vi "Measure Acoustic Frequency Response.vi"() -> ()   [LabVIEW 2022 SP3]
uses:
  <vilib>/addons/_NISVFA/_Generation/Signal Generation/SV Signal/SV Signal.lvclass/SV Signal.ctl
  <vilib>/DAQmx/write.llb/DAQmx Write (Analog Wfm 1Chan NSamp).vi
  <vilib>/DAQmx/read.llb/DAQmx Read (Analog 1D Wfm NChan NSamp).vi
  <vilib>/addons/Sound and Vibration/svt_Level/SVL AC & DC Level (Time) (1 Ch).vi
  <vilib>/addons/_NISVFA/_Generation/Signal Generation/SV Signal/Write Leading Synchronization Pulse Enable.vi
  <vilib>/addons/_NISVFA/_Generation/Signal Generation/SV Signal/Read Total Samples.vi
  <vilib>/addons/_NISVFA/_Shared subVIs/Common/svc_Get SV Channel Info.vi
  <vilib>/Analysis/baseanly.llb/Mean.vi
  <vilib>/Analysis/baseanly.llb/Mean (DBL).vi
  <vilib>/addons/_NISVFA/_Shared subVIs/Windowing/svfa_Scaled Time Domain Window (Array).vi
  <vilib>/addons/_NISVFA/_Generation/Signal Generation/SV Signal/Calculate Number of Remaining Samples.vi
  <vilib>/addons/_NISVFA/_Shared subVIs/Common/svc_Unit Label to Engineering Units.vi
  <vilib>/addons/_NISVFA/_Shared subVIs/Common/svc_Engineering Units to Unit Label.vi
  <vilib>/addons/_NISVFA/_Spectrum Processing/subVIs/svfa_Spectrum Info Window to windowTd Type Def.vi
  <vilib>/Analysis/4window.llb/Force Window.vi
  <vilib>/Analysis/4window.llb/Force Window (DBL).vi
  <vilib>/Analysis/4window.llb/Exponential Window.vi
  <vilib>/Analysis/4window.llb/Exponential Window (DBL).vi
  <vilib>/addons/_NISVFA/_Generation/Signal Generation/SV Discrete Sweep/SV Discrete Sweep.lvclass
  C:/Program Files/NI/LVAddons/nisvt/1/vi.lib/addons/_NISVFA/_Generation/Signal Generation/SV Signal/SV Signal.lvclass
  C:/Program Files/NI/LVAddons/nisvt/1/vi.lib/addons/_NISVFA/_Generation/Signal Generation/SV Function/SV Function.lvclass
  <vilib>/addons/_NISVFA/_Generation/Signal Generation/SV Discrete Sweep/Configure Frequency Sweep at Constant Amplitude.vi
  <vilib>/addons/_NISVFA/_Generation/Signal Generation/SV Signal/Write Ramp Parameters.vi
  <vilib>/addons/_NISVFA/_Generation/Signal Generation/SV Signal/Write Measurement Duration.vi
  <vilib>/addons/_NISVFA/_Generation/Signal Generation/SV Function/Write Measurement Cycles.vi
  <vilib>/addons/_NISVFA/_Generation/Signal Generation/SV Signal/Write Pre-Measurement Settling Duration.vi
  <vilib>/addons/_NISVFA/_Generation/Signal Generation/SV Function/Write Pre-Measurement Settling Cycles.vi
  <vilib>/addons/_NISVFA/_Generation/Signal Generation/SV Signal/Write Sample Rate.vi
  <vilib>/addons/_NISVFA/_Generation/Signal Generation/SV Signal/Read Generation State.vi
  <vilib>/addons/_NISVFA/_Generation/Signal Generation/SV Signal/Read System Timing Model.vi
  <vilib>/DAQmx/create/channels.llb/DAQmx Create Channel (AO-Voltage-Basic).vi
  <vilib>/DAQmx/configure/timing.llb/DAQmx Timing (Sample Clock).vi
  <vilib>/DAQmx/create/channels.llb/DAQmx Create Channel (AI-Sound Pressure-Microphone).vi
  <vilib>/DAQmx/configure/trigger.llb/DAQmx Start Trigger (Digital Edge).vi
  <vilib>/DAQmx/miscellaneous.llb/DAQmx Fill In Error Info.vi
  <vilib>/addons/_NISVFA/_Shared subVIs/Data Objects/Waveforms (DBL)/SV Read Next Measurement Data.vi
  <vilib>/addons/_NISVFA/_Shared subVIs/Common/svc_Get Window Info.vi
  <vilib>/Analysis/0measdsp.llb/Scaled Time Domain Window.vi
  <vilib>/Analysis/0measdsp.llb/Scaled Time Domain Window (DBL).vi
  <vilib>/Utility/error.llb/Error Cluster From Error Code.vi
  <vilib>/Analysis/baseanly.llb/Std Deviation and Variance.vi
  <vilib>/addons/_NISVFA/_Shared subVIs/Common/svc_Caller VI Returned in Error Source.vi
  <vilib>/addons/_NISVFA/_Spectrum Processing/SVFA Extract Single Tone Information (Waveform) (1 Ch).vi
  <vilib>/addons/_NISVFA/_Generation/Signal Generation/SV Signal/SV Signal.lvclass
  <resource>/objmgr/daqmx.rc
  <vilib>/addons/_NISVFA/_Shared subVIs/Data Objects/Waveforms (DBL)/Waveforms (N Ch).lvclass
  Program Files/NI/LVAddons/nisvt/1/examples/Sound and Vibration/SoundVib_Audio Examples.lvlib
  C:/Program Files/NI/LVAddons/nisvt/1/vi.lib/addons/_NISVFA/_Generation/Signal Generation/SV Sinusoid/SV Sinusoid.lvclass
  C:/Program Files/NI/LVAddons/nisvt/1/vi.lib/addons/_NISVFA/_Generation/Signal Generation/SV Discrete Sweep/SV Discrete Sweep.lvclass
panel:
  in  "Tab Control":enum32{"Time Domain", "Frequency Response"}(tab)=enum."Frequency Response"
  out "Waveform Graph":waveform(dbl)[](graph)=[{"t0"=timestamp(3812131384.799704 s since 1904-01-01), "dt"=1.9531249997269942e-05, "Y"=array[65939 elements], "attributes"=variant("NI_ChannelName"=variant(string "PXI1Slot2/ai0"), "NI_UnitDescription"=variant(string "Pascals"), "NI_dBReference"=variant(dbl 2e-05))}]
  out "Frequency Response":cluster{"X":dbl[], "Y":dbl[]}[](graph)=[{"X"=[10000.16250895643, 9300.551526537287, 8661.743392898796, 8076.990528350523, 7511.01433955411, 6991.165488423958, 6505.639524722646, 6059.649462837425, 5638.791827094052, 5251.483585942611, 4886.97833468438, 4567.629353940343, 4235.587558900483, 3936.8799678267396, 3676.0502040083957, 3418.4961516219546, 3182.8940845825587, 2961.9472023846033, 2757.249181768, 2566.403361400688, 2390.9470010062046, 2227.3394374433965, 2082.105166052262, 1927.4899981379963, 1795.2096498866752, 1671.116877761199, 1555.7617010555734, 1449.1771890209513, 1348.0642866026876, 1254.8715887027722, 1168.0622703473373, 1087.8906461237023, 1012.6424477531147, 942.8434270641828, 877.7564318056318, 816.9815108543755, 760.5623490709717, 708.309347567948, 659.4701187376695, 613.4296280137033, 571.3471132565072, 531.9637387870528, 495.24552739107736, 460.92109135700946, 429.09771808303145, 399.4620806680938, 371.8621259333098, 346.29727087738263, 322.46744887340316, 300.0397070573367], "Y"=[3.6256571566682783, -2.842824229562748, -0.08960303155444534, 2.249095345066365, 2.6453221558194495, 1.950185415035666, 1.243543034377954, -0.04093683877364576, 0.8379919469408734, 2.1848997103980627, 4.7478488049488305, 4.19605617553053, 5.612574046766889, 4.678952312370798, 4.014509980034741, 4.073090913593083, 4.332476772799007, 3.705298472623842, 1.6367797061942184, 4.064856703686522, 6.533918167683063, 5.093011293640562, 5.133330197154078, 4.011026255125055, 4.150393597006224, 4.30040032146349, 3.6036557635303956, 2.3710549475225817, 2.153214192355483, 2.56247383137912, 2.1421046081265924, 1.774553410980341, 0.05571083822585535, -1.5941096436671836, -1.5865003010327725, -1.8405935524517862, -1.9548534646079687, -1.8198185489247807, -1.9637495562133325, -3.3689527326194812, -3.271589837421542, -2.786050740963142, -2.6451973343748936, -2.077662686783256, -1.678738111514333, -1.682666406364262, -1.9245802060296682, -2.3869103430534615, -3.5810743320318554, -4.371652550879365]}, {"X"=[10000.16250895643, 9300.551526537287, 8661.743392898796, 8076.990528350523, 7511.01433955411, 6991.165488423958, 6505.639524722646, 6059.649462837425, 5638.791827094052, 5251.483585942611, 4886.97833468438, 4567.629353940343, 4235.587558900483, 3936.8799678267396, 3676.0502040083957, 3418.4961516219546, 3182.8940845825587, 2961.9472023846033, 2757.249181768, 2566.403361400688, 2390.9470010062046, 2227.3394374433965, 2082.105166052262, 1927.4899981379963, 1795.2096498866752, 1671.116877761199, 1555.7617010555734, 1449.1771890209513, 1348.0642866026876, 1254.8715887027722, 1168.0622703473373, 1087.8906461237023, 1012.6424477531147, 942.8434270641828, 877.7564318056318, 816.9815108543755, 760.5623490709717, 708.309347567948, 659.4701187376695, 613.4296280137033, 571.3471132565072, 531.9637387870528, 495.24552739107736, 460.92109135700946, 429.09771808303145, 399.4620806680938, 371.8621259333098, 346.29727087738263, 322.46744887340316, 300.0397070573367], "Y"=[0.014701549353104379, -0.03010901811941409, -0.0008149891758433986, -0.01724816607104709, -0.08804020536385895, 0.01171395282562733, -0.06632787060085114, -0.04128864064776648, -0.07708491466250654, -0.08538230980682754, 0.016481405604758487, -0.09831386011585251, -0.06731733883329304, -0.05245900086451385, 0.0012408175248640669, -0.07911554256372134, -0.10448091462567502, -0.03663756866557915, -0.08784017146392609, -0.08762859004910031, -0.023736243865102133, -0.0998077707827952, -0.05902392827547197, -0.14121406472839934, -0.1430330467707847, -0.1365549874396703, -0.13768685833752312, 0.05845974901477882, -0.08207883122647797, 0.034785537244882064, 0.3688104071747212, -0.05473682476494158, -0.030278179903617787, -0.13770022107713525, -0.07549590799892826, -0.04249834403098171, -0.16743475112056583, -0.20813210450439237, -0.09842685052319, -0.6864074560918922, -1.186238820840597, -0.1257540797947951, -0.040259662661179564, -0.07570918672218777, -0.10234120140370741, -0.5050386115903533, -0.6397558977539762, -0.04161640760409843, -0.07888582122962143, -2.3725881843457106]}]
  in  "sweep settings":T1(tab)=enum."EQ Settings"
  in  "speaker excitation channel":tag="PXI1Slot2/ao0"
  in  "microphone response channel":tag="PXI1Slot2/ai0"
  in  "sensor sensitivity [mV/Pa]":dbl=50.0
  in  "number of steps":i32=50 min=1
  in  "amplitude":dbl=94.0 format="%.2p dBSPL"
  in  "frequency spacing":enum16{"Linear", "Logarithmic"}(ring)=enum."Logarithmic"
  in  "sweep range":cluster{"start":dbl, "stop":dbl}={"start"=10000.0, "stop"=300.0} {"stop" min=0.0 format="%.2f"; "start" min=0.0 format="%.2f"}
  in  "output voltage ratio":dbl=3.394 format="%#_g Pa/V"
  in  "EQ Action":T2(ring)=enum."Load and Apply EQ"
  in  "EQ File":path=path "C:/dev/digital-microphone/test/EQ_test.csv"
  in  "measurement":cluster{"time":dbl, "cycles":dbl}={"time"=0.001, "cycles"=25.0} {"cycles" min=5.0 max=1000.0 step=1.0; "time" min=0.0 max=5.0 step=0.0001 format="%.3f s"}
  in  "settling":cluster{"time":dbl, "cycles":dbl}={"time"=0.0, "cycles"=1.0} {"cycles" min=0.0 max=100.0 step=0.5; "time" min=0.0 max=5.0 step=0.0001 format="%.3f s"}
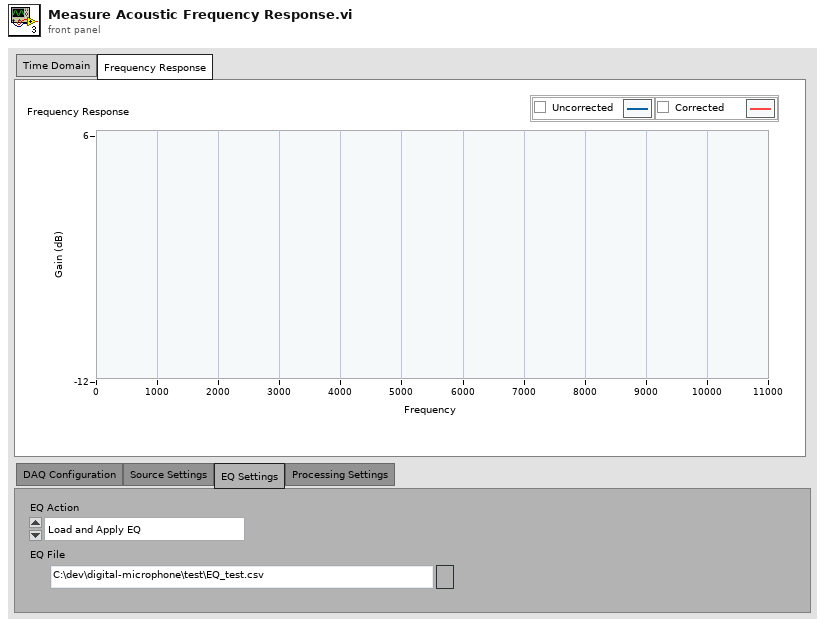
[diagram p1: front panel]
types:
  T1 = enum32{"DAQ Configuration", "Source Settings", "EQ Settings", "Processing Settings"}
  T2 = enum16{"Do Nothing", "Load and Apply EQ", "Save New EQ from Freq Response"}
  T3 = cluster{"profile":enum16{"Linear", "Half cosine"}, "durations [s]":cluster{"ramp-up":dbl, "transition":dbl, "ramp-down":dbl}}
  T4 = cluster{"frequency [Hz]":dbl, "amplitude [EU pk]":dbl, "phase (deg)":dbl}
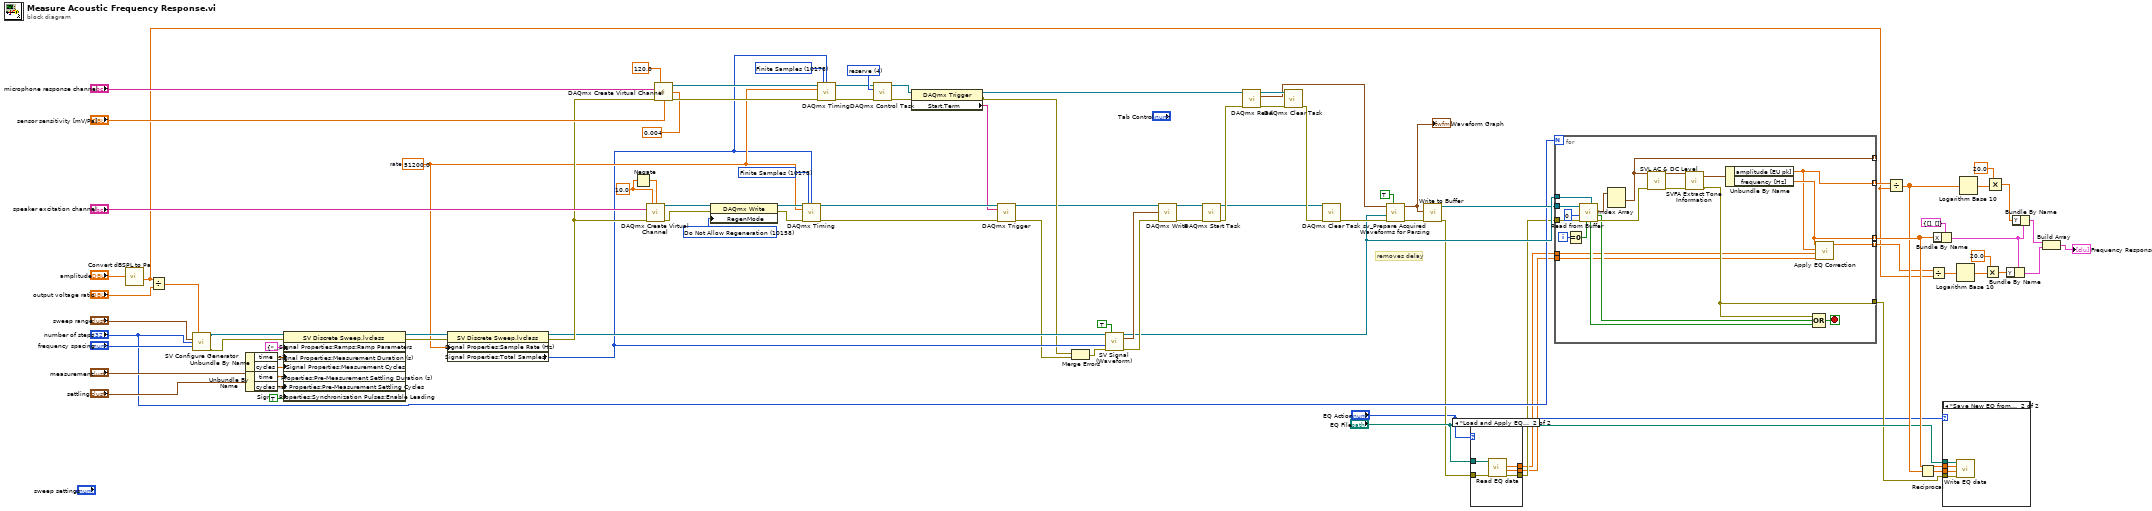
[diagram p0: block diagram]
diagram:
  w39 = 4 items=["verify"=2, "reserve"=4, "commit"=3, "unreserve"=5, "abort"=6] ("action")
  w68 = 10178 items=["Finite Samples"=10178, "Continuous Samples"=10123, "Hardware Timed Single Point"=12522] ("sample mode")
  w76 = 10158 items=["Allow Regeneration"=10097, "Do Not Allow Regeneration"=10158] ("RegenMode")
  w78 = 10.0 ("maximum value")
  w79 = 10178 items=["Finite Samples"=10178, "Continuous Samples"=10123, "Hardware Timed Single Point"=12522] ("sample mode")
  w60 = 51200.0  # rate
  # "removes delay"
  n1 = call "Convert dBSPL to Pa.vi"("dB SPL"="amplitude") -> ("Pa pk"=w7:dbl)  [unwired: 9 in, 1 out]
  n2 = Divide(x=w7, y="output voltage ratio") -> (x/y=w80:dbl)
  n3 = call-poly <vilib>:"SV Configure Generator.vi"("amplitude"=w80, "frequency range [Hz]"="sweep range", "number of steps"="number of steps", "profile"="frequency spacing") -> ("signal configuration"=w88:refnum<class "SV Discrete Sweep.lvclass">, "error out"=w87:errorcluster)  [unwired: 10 in]
  n4 = Unbundle By Name("measurement") -> ("time"=w90:dbl, "cycles"=w89:dbl)
  n5 = Unbundle By Name("settling") -> ("time"=w92:dbl, "cycles"=w91:dbl)
  n6 = property class="SV Discrete Sweep.lvclass"(reference=w88, error in=w87, "Signal Properties:Ramps:Ramp Parameters"=T3 {"profile"=enum."Half cosine", "durations [s]"={"ramp-up"=0.01, "transition"=0.0, "ramp-down"=0.01}} ("Ramp Parameters"), "Signal Properties:Measurement Duration (s)"=w90, "Signal Properties:Measurement Cycles"=w89, "Signal Properties:Pre-Measurement Settling Duration (s)"=w92, "Signal Properties:Pre-Measurement Settling Cycles"=w91, "Signal Properties:Synchronization Pulses:Enable Leading"=TRUE ("Synchronization Pulses:Enable Leading")) -> (reference out=w62:refnum<class "SV Discrete Sweep.lvclass">, error out=w63:errorcluster)
  n7 = property on="Property Node" class="SV Discrete Sweep.lvclass"(reference=w62, error in=w63, "Signal Properties:Sample Rate (Hz)"=w60) -> (reference out=w58:refnum<class "SV Discrete Sweep.lvclass">, error out=w61:errorcluster, "Signal Properties:Total Samples"=w57:i32)
  n8 = Negate(x=w78) -> (-x=w77:dbl)
  n9 = call-poly <vilib>:"DAQmx Create Virtual Channel.vi"("maximum value"=w78, "minimum value"=w77, "physical channels"="speaker excitation channel", "error in"=w61) -> ("task out"=w75:refnum<k21>, "error out"=w73:errorcluster)  [unwired: 10 in]
  n10 = call-poly <vilib>:"DAQmx Create Virtual Channel.vi"("maximum sound pressure level"=120.0, "physical channels"="microphone response channel", "current excitation value"=0.004, "error in"=w61, "microphone sensitivity"="sensor sensitivity [mV/Pa]") -> ("task out"=w70:refnum<k21>, "error out"=w69:errorcluster)  [unwired: 9 in]
  n11 = property class="DAQmx Write"(reference=w75, error in=w73, "RegenMode"=w76) -> (reference out=w74:refnum<k21>, error out=w72:errorcluster)
  n12 = call-poly <vilib>:"DAQmx Timing.vi"("task/channels in"=w74, "sample mode"=w79, "samples per channel"=w57, "rate"=w60, "error in"=w72) -> ("task out"=w55:refnum<k21>, "error out"=w53:errorcluster)  [unwired: 9 in]
  n13 = call-poly <vilib>:"DAQmx Timing.vi"("task/channels in"=w70, "sample mode"=w68, "samples per channel"=w57, "rate"=w60, "error in"=w69) -> ("task out"=w35:refnum<k21>, "error out"=w38:errorcluster)  [unwired: 9 in]
  n14 = call <vilib>:"DAQmx Control Task.vi"("task/channels in"=w35, "action"=w39, "error in"=w38) -> ("task out"=w36:refnum<k21>, "error out"=w37:errorcluster)  [unwired: 11 in]
  n15 = property on="Property Node" class="DAQmx Trigger"(reference=w36, error in=w37) -> (reference out=w42:refnum<k21>, error out=w52:errorcluster, "Start.Term"=w54:tag)
  n16 = call-poly <vilib>:"DAQmx Trigger.vi"("task/channels in"=w55, "source"=w54, "error in"=w53) -> ("task out"=w49:refnum<k21>, "error out"=w51:errorcluster)  [unwired: 11 in]
  n17 = Merge Errors(w52, w51) -> (w56:errorcluster)
  n18 = call-dynamic "SV Signal (Waveform).vi"("signal configuration"=w58, "reset"=TRUE, "samples"=w57, "error in (no error)"=w56) -> ("signal configuration"=w30:refnum<class "SV Discrete Sweep.lvclass">, "output waveform"=w48:waveform(dbl), "error out"=w50:errorcluster)  [unwired: 6 in, 3 out]
  n19 = call-poly <vilib>:"DAQmx Write.vi"("task/channels in"=w49, "data"=w48, "error in"=w50) -> ("task out"=w46:refnum<k21>, "error out"=w47:errorcluster)  [unwired: 10 in, 1 out]
  n20 = call <vilib>:"DAQmx Start Task.vi"("task/channels in"=w46, "error in"=w47) -> ("task out"=w40:refnum<k21>, "error out"=w45:errorcluster)  [unwired: 12 in]
  n21 = call-poly <vilib>:"DAQmx Read.vi"("task/channels in"=w42, "error in"=w45) -> ("task out"=w43:refnum<k21>, "data"=w32:waveform(dbl)[], "error out"=w44:errorcluster)  [unwired: 11 in]
  n22 = call <vilib>:"DAQmx Clear Task.vi"("task in"=w43, "error in"=w44) -> ("error out"=w41:errorcluster)  [unwired: 13 in]
  n23 = call <vilib>:"DAQmx Clear Task.vi"("task in"=w40, "error in"=w41) -> ("error out"=w33:errorcluster)  [unwired: 13 in]
  n24 = call "sv_Prepare Acquired Waveforms for Parsing.vi"("restart (F)"=TRUE, "error in"=w33, "SV Signal"=w30, "acquired channel waveforms"=w32) -> ("error out"=w31:errorcluster, "aligned channel waveforms"=w21:waveform(dbl)[])  [unwired: 5 in, 1 out]
  "Waveform Graph" <- w21
  n25 = call <vilib>:"Write to Buffer.vi"("error in (no error)"=w31, "waveforms"=w21) -> ("error out"=w16:errorcluster, "buffer out"=w29:refnum<data-value>)  [unwired: 7 in, 1 out]
  n26 = case shown="\"Load and Apply EQ\"" "EQ Action" {
    tunnel: "EQ File" -> [_ w99]
    tunnel: w16 -> [w94 w98]
    tunnel: [w94 w97] -> w15
    tunnel: [_ w96] -> w14
    tunnel: [_ w95] -> w13
    frame "Do Nothing", Default {
    }
    frame "Load and Apply EQ" {
      n27 = call "Read EQ data.vi"("error in (no error)"=w98, "file path"=w99) -> ("error out"=w97:errorcluster, "gain correction (x/y)"=w95:dbl[], "frequency"=w96:dbl[])  [unwired: 7 in]
    }
  }
  n28 = for {
    N: "number of steps" -> [_]
    tunnel: w29 -> [w117]
    tunnel: w30 -> [w116]
    tunnel: w15 -> [w115]
    tunnel: [w104] -> w20 mode=indexing
    tunnel: [w111] -> _ mode=indexing
    tunnel: [w103] -> w26 mode=indexing
    tunnel: w14 -> [w102]
    tunnel: w13 -> [w101]
    tunnel: [w105] -> w12
    tunnel: [w100] -> w8 mode=indexing
    i -> [w110]
    stop <- w112 stop-if-true
    n29 = Equal To 0?(x=w110) -> (x = 0?=w109:bool)
    n30 = call-poly <vilib>:"Read from Buffer.vi"("test signal configuration"=w116, "reset start (F)"=w109, "error in (no error)"=w115, "timeout (1000 ms)"=0, "buffer"=w117) -> ("error out"=w120:errorcluster, "end of buffer"=w113:bool, "waveforms subset"=w114:waveform(dbl)[], "done"=w119:bool)  [unwired: 2 in, 1 out]
    n31 = Index Array(array=w114) -> (element #1=w111:waveform(dbl))  [unwired: 2 in, 1 out]
    n32 = call-poly <vilib>:"SVL AC & DC Level.vi"("scaled signal [EU]"=w111, "error in (no error)"=w120) -> ("AC signal [EU]"=w108:waveform(dbl), "error out"=w107:errorcluster)  [unwired: 12 in, 4 out]
    n33 = call-poly <vilib>:"SVFA Extract Tone Information.vi"("scaled signal [EU]"=w108, "error in"=w107) -> ("detected tone"=w106:T4, "error out"=w105:errorcluster)  [unwired: 15 in, 1 out]
    n34 = Unbundle By Name(w106) -> ("amplitude [EU pk]"=w103:dbl, "frequency [Hz]"=w104:dbl)
    n35 = Compound Arithmetic op=OR(w105, w113, w119) -> (w112:bool)
    n36 = call "Apply EQ Correction.vi"("gain correction (x/y)"=w101, 9:"frequency"=w102, "amplitude"=w103, 11:"frequency"=w104) -> ("corrected amplitude"=w100:dbl)  [unwired: 7 in]
  }
  n37 = Divide(x=w26, y=w7) -> (x/y=w19:dbl[])
  n38 = Reciprocal(x=w19) -> (1/x=w18:dbl[])
  n39 = Divide(x=w8, y=w7) -> (x/y=w9:dbl[])
  n40 = Bundle By Name(cluster=cluster{"X":dbl[], "Y":dbl[]} {"X"=[], "Y"=[]} ("THD vs Amplitude"), "X"=w20) -> (w5:cluster{"X":dbl[], "Y":dbl[]})
  n41 = case shown="\"Save New EQ from Freq Response\"" "EQ Action" {
    tunnel: w20 -> [_ w124]
    tunnel: w18 -> [_ w123]
    tunnel: "EQ File" -> [_ w122]
    tunnel: w12 -> [_ w121]
    frame "Do Nothing", Default {
    }
    frame "Save New EQ from Freq Response" {
      n42 = call "Write EQ data.vi"("error in (no error)"=w121, "gain correction (x/y)"=w123, "frequency"=w124, "file path"=w122) -> ()  [unwired: 7 in, 1 out]
    }
  }
  n43 = Logarithm Base 10(1:w9) -> (0:w11:dbl[])
  n44 = Logarithm Base 10(1:w19) -> (0:w25:dbl[])
  n45 = Multiply(x=20.0, y=w11) -> (x*y=w6:dbl[])
  n46 = Multiply(x=20.0, y=w25) -> (x*y=w24:dbl[])
  n47 = Bundle By Name(cluster=w5, "Y"=w6) -> (w4:cluster{"X":dbl[], "Y":dbl[]})
  n48 = Bundle By Name(cluster=w5, "Y"=w24) -> (w3:cluster{"X":dbl[], "Y":dbl[]})
  n49 = Build Array(w3, w4) -> (→"Frequency Response":cluster{"X":dbl[], "Y":dbl[]}[])
